vi "sendTelFromTcpClient.vi"(8 "error in (no error)":errorcluster, 10 "tel connection ID in":refnum<k5>, 11 "TcpServer in":refnum<class "TcpServer.lvclass">) -> (0 "error out":errorcluster, 2 "tel connection ID out":refnum<k5>, 3 "TcpServer out":refnum<class "TcpServer.lvclass">)   [LabVIEW 2018]
doc: "Send an element to the TCP server."
uses:
  src/TcpServer/TcpServer.lvclass
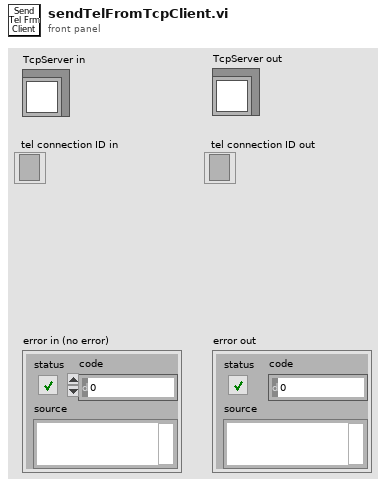
[diagram p1: front panel]
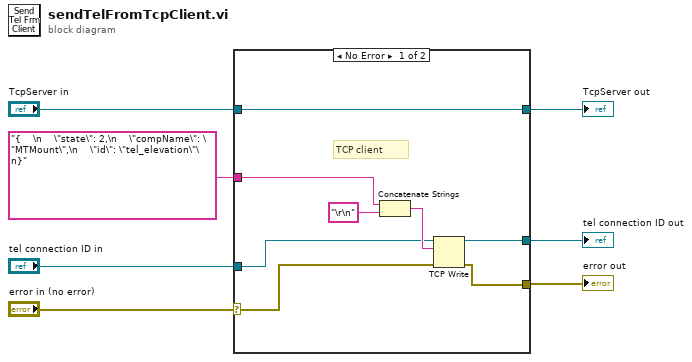
[diagram p0: block diagram]
diagram:
  n1 = case shown="No Error" "error in (no error)" {
    selector: "error in (no error)" -> [w13 w18]
    tunnel: [w14 w16] -> w7
    tunnel: [w15 w17] -> w6
    tunnel: "TcpServer in" -> [w14 w16]
    tunnel: [w11 w18] -> w3
    tunnel: "tel connection ID in" -> [w10 w17]
    tunnel: "{    \n    \"state\": 2,\n    \"compName\": \"MTMount\",\n    \"id\": \"tel_elevation\"\n}" ("Display") -> [w9 _]
    frame No Error {
      # "TCP client"
      n2 = Concatenate Strings(w9, "\r\n" ("string")) -> (w12:string)
      n3 = TCP Write(connection ID=w10, data in=w12, error in (no error)=w13) -> (connection ID out=w15:refnum<k5>, error out=w11:errorcluster)  [unwired: 1 in, 1 out]
    }
    frame Error {
    }
  }
  "TcpServer out" <- w7
  "tel connection ID out" <- w6
  "error out" <- w3
